vi "midi_InstrumentDefinition.vi"(10 "fs (Hz)":dbl, 11 "note":dbl[](array[numeric])) -> (3 "audio":dbl[](array[numeric]))   [LabVIEW 2013]
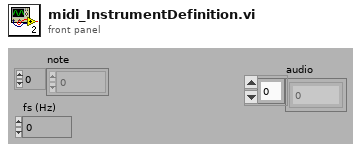
[diagram p1: front panel]
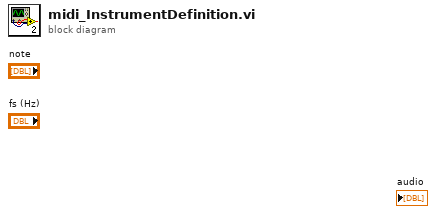
[diagram p0: block diagram]
diagram:
